vi "Create MyAccess Database.vi"() -> ()   [LabVIEW 2014]
panel:
  in  "路径":path=path "D:/MyAccessDB.mdb" caption="ACCESS数据库MDB文件"
  out "错误输出":errorcluster
  in  "ADOX._Catalog":refnum<k7>
  # "使用ActiveX命令来创建新的Access数据库文件。\n     1.从ActiveX面板选择Automation Open VI打开一个\"Microsoft ADO Ext. x.x for DDL and Security Version x.x\"引用，其中x.x 代表版本号。 \n     2.右键单击选择Catalog对象。 \n     3.在程序框图放置一个方法节点并将之连接至Automation Open函数。右键单击 Method?Select Method选择Create方法。 \n     4.右键点击参数 Connect String输入选择 Create?Constant。输入字符串常量：Provider=Microsoft.Jet.OLEDB.4.0;Data Source=yourfilename.mdb。 文件名是创建的Access数据库文件路径名，譬如C:\\My Documents\\MyAccessDB.mdb。"
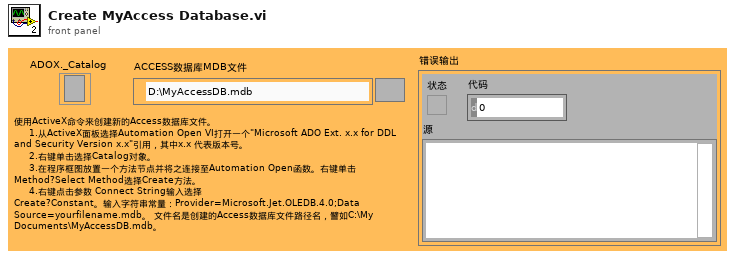
[diagram p1: front panel]
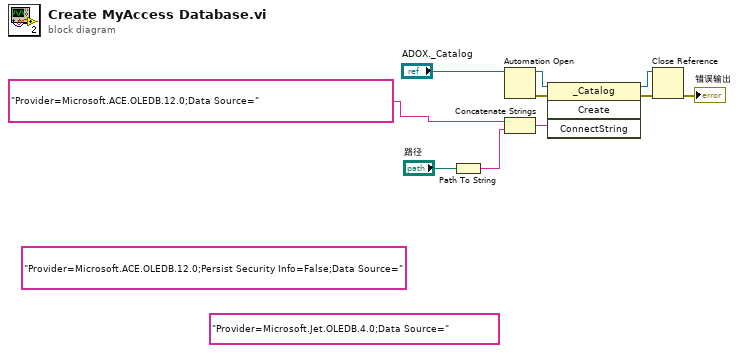
[diagram p0: block diagram]
diagram:
  (unwired) "Provider=Microsoft.ACE.OLEDB.12.0;Persist Security Info=False;Data Source=" ("ConnectString")
  (unwired) "Provider=Microsoft.Jet.OLEDB.4.0;Data Source=" ("ConnectString")
  n1 = Path To String(path="路径") -> (string=w3:string)
  n2 = Automation Open ("打开自动化")(Automation Refnum="ADOX._Catalog") -> (Automation Refnum=w9:refnum<k7>, error out=w7:errorcluster)  [unwired: 3 in]
  n3 = Concatenate Strings("Provider=Microsoft.ACE.OLEDB.12.0;Data Source=" ("ConnectString"), w3) -> (w2:string)
  n4 = invoke class="_Catalog" method="Create"(reference=w9, error in=w7, "ConnectString"=w2) -> (reference out=w8:refnum<k7>, error out=w6:errorcluster)  [unwired: 1 in, 2 out]
  n5 = Close Reference(reference=w8, error in (no error)=w6) -> (error out=→"错误输出":errorcluster)
